vi "Check mtcdt check thumb drive write test.vi"(6 "VISA resource name":refnum<visa-resource-name>="COM5", 7 "Passed so far":bool, 8 "error in (no error)":errorcluster) -> (0 "error out":errorcluster, 1 "Card response":string, 2 "Source Response":string, 4 "VISA Refnum out":refnum<visa-resource-name>, 5 "Passed?":bool)   [LabVIEW 2024]
panel:
  out "dest cksum":string
  out "src cksum":string
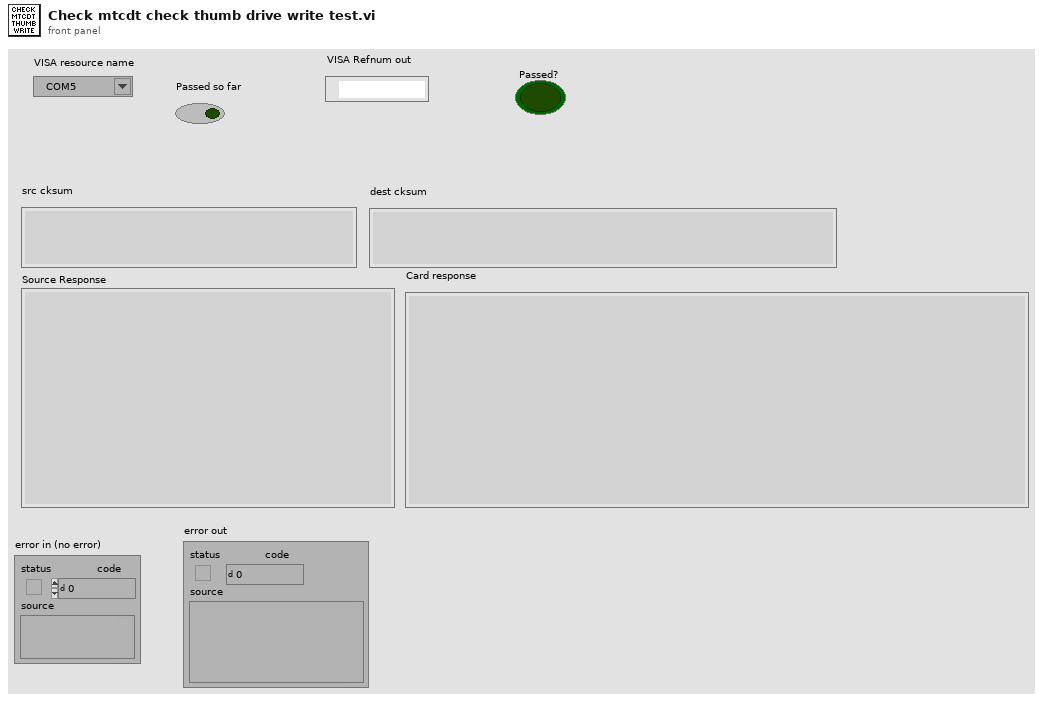
[diagram p1: front panel]
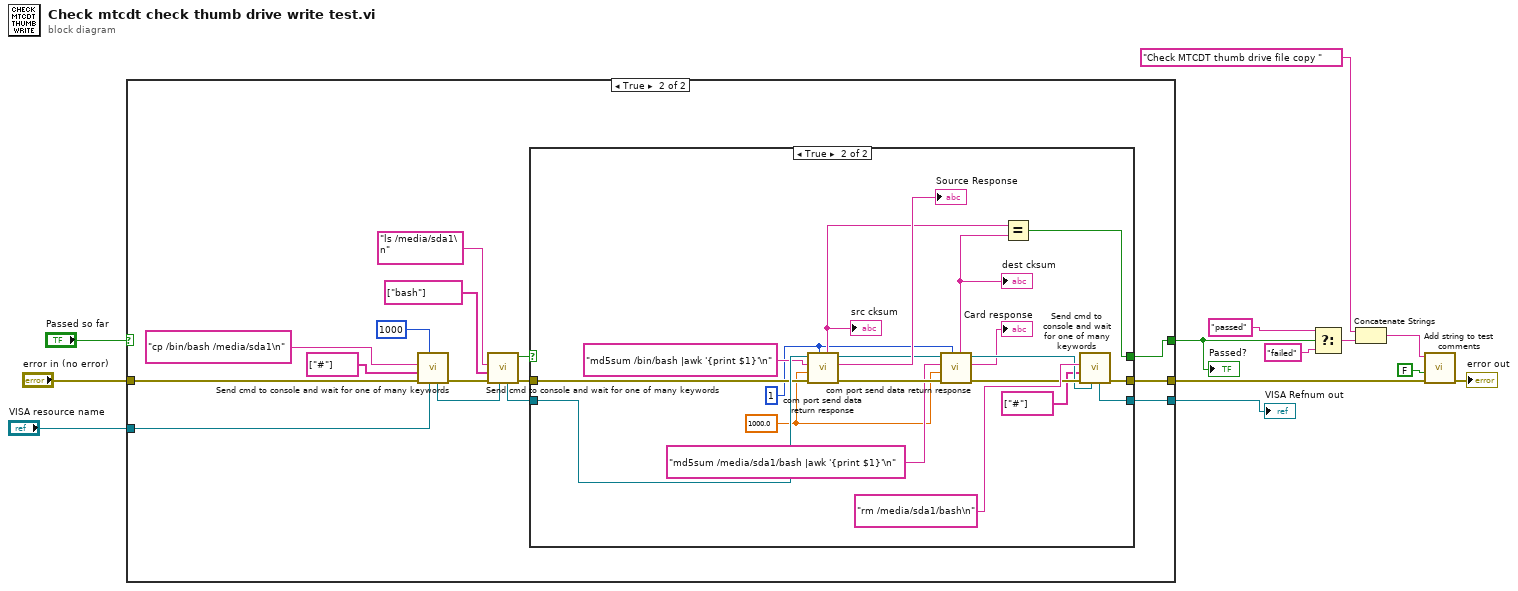
[diagram p0: block diagram]
diagram:
  n1 = case shown="True" "Passed so far" {
    selector: "Passed so far" -> [w16 _]
    tunnel: "error in (no error)" -> [w15 w31]
    tunnel: [w15 w19] -> w1
    tunnel: "VISA resource name" -> [w14 w29]
    tunnel: [w16 w18] -> w5
    tunnel: [w14 w20] -> w2
    frame False {
    }
    frame True {
      n2 = call "Send cmd to console and wait for one of many keywords.vi"("VISA resource name"=w29, "Timeout (1000 mSecs)"=u32 1000 ("Timeout (mSecs)"), "error in (no error)"=w31, "Wait for keywords"=string[] ["#"], "cmd"="cp /bin/bash /media/sda1\n") -> ("error out"=w17:errorcluster, "VISA Refnum out"=w26:refnum<visa-resource-name>)  [unwired: 2 in, 3 out]
      n3 = call "Send cmd to console and wait for one of many keywords.vi"("VISA resource name"=w26, "error in (no error)"=w17, "Wait for keywords"=string[] ["bash"], "cmd"="ls /media/sda1\n" ("write buffer")) -> ("error out"=w22:errorcluster, "Found key?"=w23:bool, "VISA Refnum out"=w21:refnum<visa-resource-name>)  [unwired: 3 in, 2 out]
      n4 = case shown="True" w23 {
        selector: w23 -> [w32 _]
        tunnel: w22 -> [w34 w48]
        tunnel: w21 -> [w33 w49]
        tunnel: [w34 w52] -> w19
        tunnel: [w32 w51] -> w18
        tunnel: [w33 w50] -> w20
        frame False {
        }
        frame True {
          w40 = u32 1 ("Return line number")
          w42 = 1000.0 ("Wait Msecs for response")
          n5 = call "com port send data return response.vi"("Return line number"=w40, "error in (no error)"=w48, "Wait Msecs for response"=w42, "Send data"="md5sum /bin/bash |awk '{print $1}'\n", "VISA resource name"=w49) -> ("error out"=w45:errorcluster, "response"=→"Source Response":string, "VISA resource name out"=w44:refnum<visa-resource-name>, "Response Line"=w41:string)  [unwired: 2 in, 1 out]
          "src cksum" <- w41
          n6 = call "com port send data return response.vi"("Return line number"=w40, "error in (no error)"=w45, "Wait Msecs for response"=w42, "Send data"="md5sum /media/sda1/bash |awk '{print $1}'\n", "VISA resource name"=w44) -> ("error out"=w38:errorcluster, "response"=→"Card response":string, "VISA resource name out"=w37:refnum<visa-resource-name>, "Response Line"=w39:string)  [unwired: 2 in, 1 out]
          "dest cksum" <- w39
          n7 = Equal?(x=w41, y=w39) -> (x = y?=w51:bool)
          n8 = call "Send cmd to console and wait for one of many keywords.vi"("VISA resource name"=w37, "error in (no error)"=w38, "Wait for keywords"=string[] ["#"], "cmd"="rm /media/sda1/bash\n" ("write buffer")) -> ("error out"=w52:errorcluster, "VISA Refnum out"=w50:refnum<visa-resource-name>)  [unwired: 3 in, 3 out]
        }
      }
    }
  }
  "Passed?" <- w5
  "VISA Refnum out" <- w2
  n9 = Select(t="passed", s=w5, f="failed") -> (s? t:f=w9:string)
  n10 = Concatenate Strings("Check MTCDT thumb drive file copy " ("string"), w9) -> (w8:string)
  n11 = call "Add string to test comments.vi"("error in (no error)"=w1, "New Section (y)?"=FALSE, "Comments"=w8) -> ("error out"=→"error out":errorcluster)  [unwired: 7 in, 1 out]
